vi "Format LVXML_GetTagValue.vi"(8 "error in (no error)":errorcluster, 10 "xmlDataIn":T2, 11 "Tag name":string) -> (0 "error out":errorcluster, 2 "Value":string, 3 "xmlDataOut":T2)   [LabVIEW 2014, in "AWS_EC2.lvlib" / "AWS_EC2.lvclass"]
uses:
  AWS_EC2.lvclass
  lv-xml-parser/r0/trunk/VI Source/EventType.ctl
  lv-xml-parser/r0/trunk/VI Source/LV XML Parser.lvlib
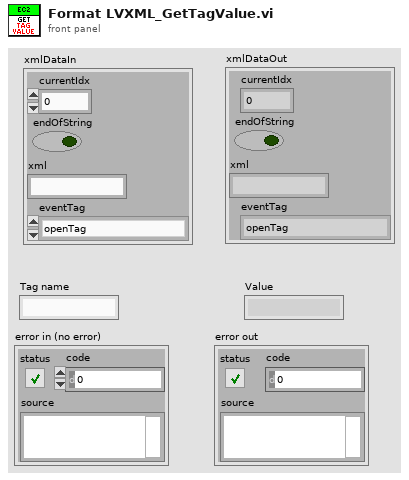
[diagram p1: front panel]
types:
  T1 = typedef "LV XML Parser.lvlib/EventType.ctl" = enum16{"openTag", "endOpenTag", "closeTag", "comment", "endComment", "endOfFile", "attribute", "startXml"}
  T2 = cluster{"currentIdx":i32, "endOfString":bool, "xml":string, "eventTag":T1}
  T3 = cluster{"namespaceUri":string, "localName":string}
  T4 = cluster{"Attributes":cluster{"localName":string, "namespaceUri":string, "value":string}[], "localName":string, "namespaceUri":string, "valueXmlData":cluster{"currentIdx":i32, "endOfString":bool, "xml":string, "eventTag":T1}}[]
  T5 = cluster{"Attributes":cluster{"localName":string, "namespaceUri":string, "value":string}[], "localName":string, "namespaceUri":string, "valueXmlData":cluster{"currentIdx":i32, "endOfString":bool, "xml":string, "eventTag":T1}}
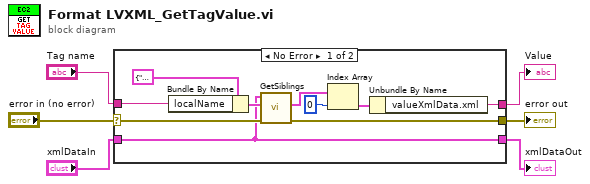
[diagram p0: block diagram]
diagram:
  n1 = case shown="No Error" "error in (no error)" {
    selector: "error in (no error)" -> [w8 w18]
    tunnel: [w16 _] -> w6
    tunnel: [w15 w18] -> w5
    tunnel: "Tag name" -> [w10 _]
    tunnel: "xmlDataIn" -> [w7 w17]
    tunnel: [w7 w17] -> w1
    frame No Error {
      n2 = Bundle By Name(cluster=T3 {"namespaceUri"="", "localName"=""} ("limitToTag"), "localName"=w10) -> (w11:T3)
      n3 = call "GetSiblings.vi"("error in (no error)"=w8, "limitToTag"=w11, "xmlData"=w7) -> ("error out"=w15:errorcluster, "Siblings"=w12:T4)  [unwired: 7 in]
      n4 = Index Array(array=w12, index=0) -> (element=w14:T5)
      n5 = Unbundle By Name(w14) -> ("valueXmlData.xml"=w16:string)
    }
    frame Error {
    }
  }
  "Value" <- w6
  "error out" <- w5
  "xmlDataOut" <- w1
